vi "Periodic Tasks.vi"(8 "error in":errorcluster) -> ()   [LabVIEW 2019]
doc: "This VI runs in parallel to other tasks. It can contain as many user-defined periodic loops as you need. These can carry out PID or other sorts of timed response."
uses:
  <vilib>/Rock Robotics/WPI/Relay/WPI_RelayValue.ctl
  <vilib>/Rock Robotics/WPI/ThirdParty/Phoenix-LabVIEW/Motor Controller/Controls/CTRE_Phoenix_MotorControl_ControlMode.ctl
  <vilib>/Rock Robotics/WPI/Solenoid/WPI_SolenoidValue.ctl
  Robot Global Data.vi
  <vilib>/Rock Robotics/WPI/Solenoid/WPI_SolenoidSetEnum.vi
panel:
  in  "Proportional":dbl
  in  "Integral":dbl
  in  "Derivative":dbl
  in  "slotIdx":i32
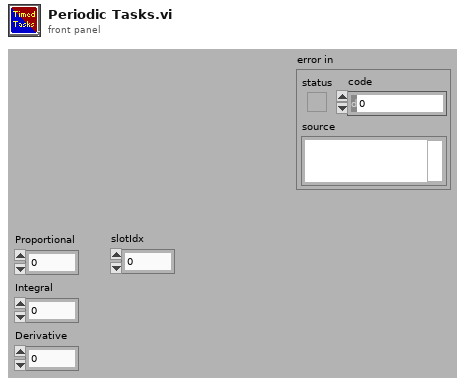
[diagram p1: front panel]
types:
  T1 = typedef "WPI_MotorControlDeviceRef.ctl" = cluster{"DeviceStatus":errorcluster, "Type":T2, "PWM":cluster{"PWM Channel":T3, "DeadBand":T4}, "CAN":cluster{"Device Number":u8, "SetOutput VI Ref":variant, "GetOutput VI Ref":variant, "Enable VI Ref":variant, "Disable VI Ref":variant, "Data":variant}, "Invert":bool, "DIO PWM":cluster{"PWM \"Enable\" Channel":T3, "DIOChannel":T5, "PWM Rate":dbl}}
  T2 = typedef "WPI_MotorControlType.ctl" = enum16{"PWM", "CAN", "DIO PWM"}
  T3 = typedef "FPGA_DIOPWMChannel.ctl" = enum8{"PWM 0", "PWM 1", "PWM 2", "PWM 3", "PWM 4", "PWM 5", "PWM 6", "PWM 7", "PWM 8", "PWM 9", "PWM MXP 0", "PWM MXP 1", "PWM MXP 2", "PWM MXP 3", "PWM MXP 4", "PWM MXP 5", "PWM MXP 6", "PWM MXP 7", "PWM MXP 8", "PWM MXP 9", "Invalid"}
  T4 = typedef "WPI_PWMDeadband.ctl" = cluster{"Name":string, "maxPositivePwm":i32, "minPositivePwm":i32, "centerPwm":i32, "maxNegativePwm":i32, "minNegativePwm":i32, "angularRange":u16}
  T5 = typedef "FPGA_DIOChannel.ctl" = enum8{"DIO 0", "DIO 1", "DIO 2", "DIO 3", "DIO 4", "DIO 5", "DIO 6", "DIO 7", "DIO 8", "DIO 9", "DIO MXP 0", "DIO MXP 1", "DIO MXP 2", "DIO MXP 3", "DIO MXP 4", "DIO MXP 5", "DIO MXP 6", "DIO MXP 7", "DIO MXP 8", "DIO MXP 9", "DIO MXP 10", "DIO MXP 11", "DIO MXP 12", "DIO MXP 13", "DIO MXP 14", "DIO MXP 15", "SPI Port CS1", "SPI Port CS2", "SPI Port CS3", "SPI Port MISO", "SPI Port MOSI", "Invalid"}
  T6 = typedef "WPI_SolenoidDevRef.ctl" = cluster{"DevStatus":errorcluster, "Pneumatics Control Module":u8, "Forward Solenoid Channel":T7, "Reverse Solenoid Channel":T7}
  T7 = typedef "WPI_SolenoidChannel.ctl" = enum8{"Solenoid 0", "Solenoid 1", "Solenoid 2", "Solenoid 3", "Solenoid 4", "Solenoid 5", "Solenoid 6", "Solenoid 7", "Invalid"}
  T8 = typedef "WPI_AnalogChannelDevRef.ctl" = cluster{"DevStatus":errorcluster, "Analog Channel":T9}
  T9 = typedef "FPGA_AIChannel.ctl" = enum8{"AI 0", "AI 1", "AI 2", "AI 3", "AI MXP 0", "AI MXP 1", "AI MXP 2", "AI MXP 3", "Invalid"}
  T10 = typedef "WPI_RelayDevRef.ctl" = cluster{"DevStatus":errorcluster, "Relay Channel":T11, "Relay Direction":T12}
  T11 = typedef "FPGA_DIORelayChannel.ctl" = enum8{"Relay 0", "Relay 1", "Relay 2", "Relay 3", "Invalid"}
  T12 = typedef "WPI_RelayDirection.ctl" = enum16{"Both directions", "Forward only", "Reverse only"}
  T13 = typedef "WPI_RelayValue.ctl" = enum16{"Off", "On", "Forward", "Reverse"}
  T14 = enum16{"DemandType_Neutral", "DemandType_AuxPID", "DemandType_ArbitraryFeedForward"}
  T15 = typedef "WPI_SolenoidValue.ctl" = enum16{"Off", "On", "Forward", "Reverse"}
  T16 = typedef "CTRE_Phoenix_MotorControl_ControlMode.ctl" = u16
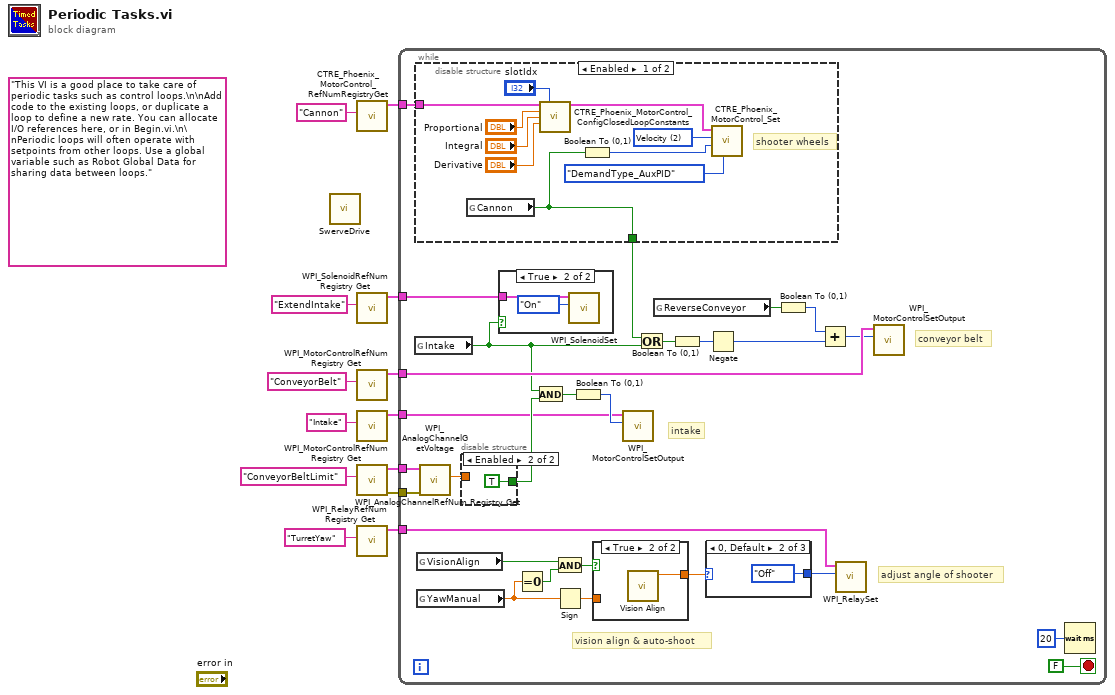
[diagram p0: block diagram]
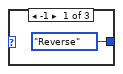
[diagram p2: hidden frame]
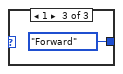
[diagram p3: hidden frame]
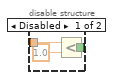
[diagram p4: hidden frame]
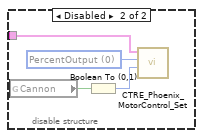
[diagram p5: hidden frame]
diagram:
  (unwired) "This VI is a good place to take care of periodic tasks such as control loops.\n\nAdd code to the existing loops, or duplicate a loop to define a new rate. You can allocate I/O references here, or in Begin.vi.\n\nPeriodic loops will often operate with setpoints from other loops. Use a global variable such as Robot Global Data for sharing data between loops."
  n1 = call "SwerveDrive.vi"() -> ()  [unwired: 12 in]
  n2 = call <vilib>:"CTRE_Phoenix_MotorControl_RefNumRegistryGet.vi"("refnum name"="Cannon") -> ("PhoenixMotorControlDevRef"=w5:T1)  [unwired: 9 in, 1 out]
  n3 = call <vilib>:"WPI_SolenoidRefNum Registry Get.vi"("refnum name"="ExtendIntake") -> ("SolenoidDevRef"=w9:T6)  [unwired: 9 in, 1 out]
  n4 = call <vilib>:"WPI_MotorControlRefNum Registry Get.vi"("refnum name"="ConveyorBelt") -> ("MotorControlDevRef"=w1:T1)  [unwired: 9 in, 1 out]
  n5 = call <vilib>:"WPI_MotorControlRefNum Registry Get.vi"("refnum name"="Intake") -> ("MotorControlDevRef"=w7:T1)  [unwired: 9 in, 1 out]
  n6 = call <vilib>:"WPI_AnalogChannelRefNum Registry Get.vi"("refnum name"="ConveyorBeltLimit") -> ("error out"=w12:errorcluster, "AIDeviceRef"=w11:T8)  [unwired: 9 in]
  n7 = call <vilib>:"WPI_RelayRefNum Registry Get.vi"("refnum name"="TurretYaw") -> ("RelayDevRef"=w3:T10)  [unwired: 9 in, 1 out]
  n8 = while {
    tunnel: w12 -> [w32]
    tunnel: w11 -> [w31]
    tunnel: w9 -> [w30]
    tunnel: w7 -> [w24]
    tunnel: w5 -> [w29]
    tunnel: w3 -> [w28]
    tunnel: w1 -> [w22]
    stop <- FALSE stop-if-true
    # "adjust angle of shooter"
    # "conveyor belt"
    # "intake"
    # "vision align & auto-shoot"
    n9 = global read "Robot Global Data.vi" "Intake"() -> (w21:bool)
    n10 = disable-structure shown="Enabled" {
      disable-tunnel: w29 -> [w58 w62]
      disable-tunnel: [w50 _] -> w25
      frame Enabled {
        w55 = T16 2 items=["PercentOutput"=0, "Position"=1, "Velocity"=2, "Current"=3, "Follower"=5, "MotionProfile"=6, "MotionMagic"=7, "MotionProfileArc"=10, "Disabled"=15] ("Control Mode")
        # "shooter wheels"
        n11 = global read "Robot Global Data.vi" "Cannon"() -> (w50:bool)
        n12 = call <vilib>:"CTRE_Phoenix_MotorControl_ConfigClosedLoopConstants.vi"("PhoenixMotorControlDevRef"=w58, "slotIdx"="slotIdx", "P"="Proportional", "I"="Integral", "D"="Derivative") -> ("PhoenixMotorControlDevRef"=w56:T1)  [unwired: 9 in, 1 out]
        n13 = Boolean To (0,1)(Boolean=w50) -> (0, 1=w49:i16)
        n14 = call <vilib>:"CTRE_Phoenix_MotorControl_Set.vi"("DemandType"=T14."DemandType_AuxPID", "Output"=w49, "Control Mode"=w55, "PhoenixMotorControlDevRef"=w56) -> ()  [unwired: 6 in, 2 out]
      }
      frame Disabled {
        w61 = T16 0 items=["PercentOutput"=0, "Position"=1, "Velocity"=2, "Current"=3, "Follower"=5, "MotionProfile"=6, "MotionMagic"=7, "MotionProfileArc"=10, "Disabled"=15] ("Control Mode")
        n15 = global read "Robot Global Data.vi" "Cannon"() -> (w60:bool)
        n16 = Boolean To (0,1)(Boolean=w60) -> (0, 1=w59:i16)
        n17 = call <vilib>:"CTRE_Phoenix_MotorControl_Set.vi"("Output"=w59, "Control Mode"=w61, "PhoenixMotorControlDevRef"=w62) -> ()  [unwired: 7 in, 2 out]
      }
    }
    n18 = global read "Robot Global Data.vi" "VisionAlign"() -> (w37:bool)
    n19 = global read "Robot Global Data.vi" "YawManual"() -> (w36:dbl)
    n20 = call <vilib>:"WPI_AnalogChannelGetVoltage.vi"("error in (no error)"=w32, "AIDeviceRef"=w31) -> ("Voltage"=w33:dbl)  [unwired: 7 in, 2 out]
    n21 = disable-structure shown="Enabled" {
      disable-tunnel: w33 -> [w47 _]
      disable-tunnel: [w45 TRUE] -> w26
      frame Disabled {
        n22 = Less?(x=w47, y=1.0) -> (x < y?=w45:bool)
      }
      frame Enabled {
      }
    }
    n23 = case shown="True" w21 {
      tunnel: w30 -> [_ w64]
      frame False {
      }
      frame True {
        n24 = call-poly <vilib>:"WPI_SolenoidSet.vi"("Value"=WPI_SolenoidValue."On", "SolenoidDevRef"=w64) -> ()  [unwired: 8 in, 2 out]
      }
    }
    n25 = Equal To 0?(x=w36) -> (x = 0?=w35:bool)
    n26 = And(x=w21, y=w26) -> (x .and. y?=w23:bool)
    n27 = And(x=w37, y=w35) -> (x .and. y?=w38:bool)
    n28 = Sign(1:w36) -> (0:w18:dbl)
    n29 = Boolean To (0,1)(Boolean=w23) -> (0, 1=w39:i16)
    n30 = case shown="True" w38 {
      tunnel: w18 -> [w65 _]
      tunnel: [w65 w66] -> w19
      frame False {
      }
      frame True {
        n31 = call "Vision Align.vi"() -> ("YawAdjustment"=w66:dbl)  [unwired: 11 in]
      }
    }
    n32 = call <vilib>:"WPI_MotorControlSetOutput.vi"("Output"=w39, "MotorControlDevRef"=w24) -> ()  [unwired: 7 in, 3 out]
    n33 = Or(x=w25, y=w21) -> (x .or. y?=w27:bool)
    n34 = global read "Robot Global Data.vi" "ReverseConveyor"() -> (w17:bool)
    n35 = Boolean To (0,1)(Boolean=w27) -> (0, 1=w34:i16)
    n36 = case shown="0, Default" w19 {
      tunnel: [WPI_RelayValue."Reverse" ("YawAdjustment") WPI_RelayValue."Off" ("YawAdjustment") WPI_RelayValue."Forward" ("YawAdjustment")] -> w20
      frame -1 {
      }
      frame 0, Default {
      }
      frame 1 {
      }
    }
    n37 = Negate(x=w34) -> (-x=w15:i16)
    n38 = Boolean To (0,1)(Boolean=w17) -> (0, 1=w16:i16)
    n39 = Add(x=w16, y=w15) -> (x+y=w14:i16)
    n40 = call <vilib>:"WPI_RelaySet.vi"("RelayValue"=w20, "RelayDevRef"=w28) -> ()  [unwired: 8 in, 2 out]
    n41 = call <vilib>:"WPI_MotorControlSetOutput.vi"("Output"=w14, "MotorControlDevRef"=w22) -> ()  [unwired: 7 in, 3 out]
    n42 = Wait (ms)(milliseconds to wait=u32 20) -> ()  [unwired: 1 out]
  }
